vi "Configure Expected Nominal Power.vi"(8 "error in (no error)":errorcluster, 9 "Expected Nominal Power (3.500000E+01)":dbl=35.0 format="%^.3e", 10 "Instance (1)":i32=1, 11 "VISA resource name":refnum<visa-resource-name>) -> (0 "error out":errorcluster, 3 "VISA resource name out":refnum<visa-resource-name>)   [LabVIEW 2020, in "Rohde&Schwarz CMP LR WPAN Measurement.lvlib"]
doc: "Sets the expected nominal power of the measured RF signal.\n\nAttribute:\nRSCMPLRWM_ATTR_EXPECTED_NOMINAL_POWER\n\nRemote-control command:\nCONFigure:WPAN:MEAS<i>:RFSettings:ENPower"
uses:
  <instrlib>/Rohde&Schwarz CMP LR WPAN Measurement/Rohde&Schwarz CMP LR WPAN Measurement.lvlib
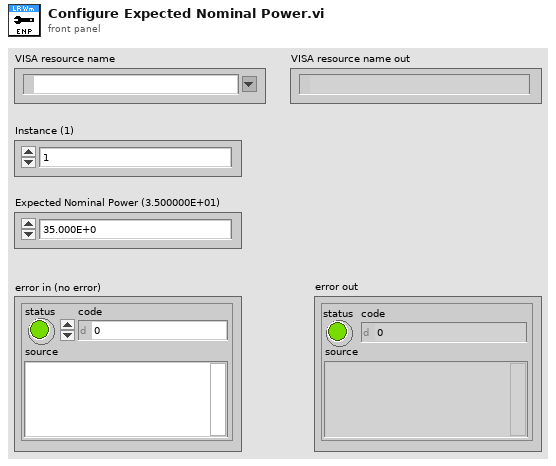
[diagram p1: front panel]
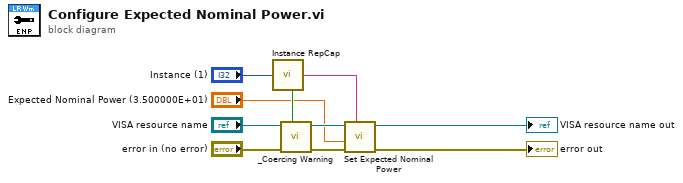
[diagram p0: block diagram]
diagram:
  n1 = call <instrlib>:"Instance RepCap.vi"("Instance In"="Instance (1)") -> ("In Range?"=w3:bool, "RepCap Identifier Out"=w8:string)  [unwired: 1 in]
  n2 = call <instrlib>:"_Coercing Warning.vi"("In Range?"=w3, "error in (no error)"="error in (no error)", "VISA resource name"="VISA resource name") -> ("error out"=w5:errorcluster, "VISA resource name out"=w4:refnum<visa-resource-name>)  [unwired: 7 in]
  n3 = call "Set Expected Nominal Power"("Repeated Capabilities"=w8, "error in (no error)"=w5, "Expected Nominal Power (0.0)"="Expected Nominal Power (3.500000E+01)", "instrument handle"=w4) -> ("error out"=→"error out":errorcluster, "instrument handle out"=→"VISA resource name out":refnum<visa-resource-name>)  [unwired: 6 in]
